vi "Close.vi"(8 "error in (no error)":errorcluster, 11 "DiscoveryService in":refnum<class "NodeDiscovery.lvclass">) -> (0 "error out":errorcluster)   [LabVIEW 2020, in "Vecto.lvlib" / "NodeDiscovery.lvclass"]
uses:
  NodeDiscovery.lvclass
  NodeDiscovery.lvclass/NodeDiscovery.ctl
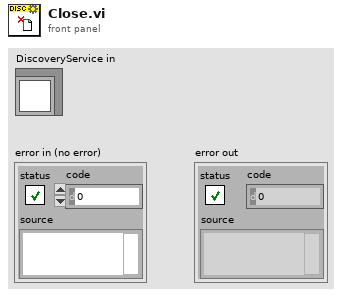
[diagram p1: front panel]
types:
  T1 = typedef "Vecto.lvlib/NodeDiscovery.lvclass/Incoming Events.ctl" = cluster{"Close":refnum<user-event>, "Update Service":refnum<user-event>, "Update Status":refnum<user-event>, "Remove Service":refnum<user-event>}
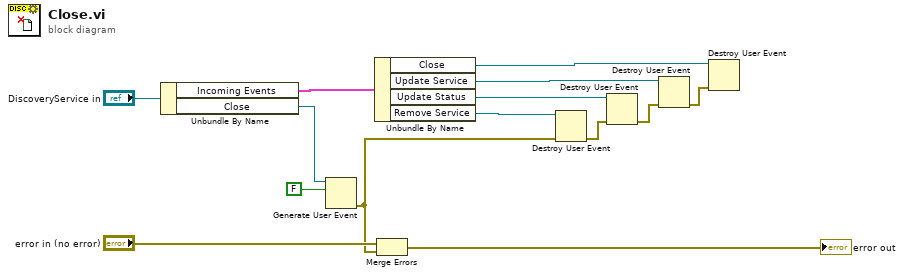
[diagram p0: block diagram]
diagram:
  n1 = Unbundle By Name("DiscoveryService in") -> ("Incoming Events"=w11:T1, "Close"=w13:refnum<user-event>)
  n2 = Generate User Event(user event=w13, event data cluster=FALSE ("event data")) -> (error out=w1:errorcluster)  [unwired: 2 in, 1 out]
  n3 = Unbundle By Name(w11) -> ("Close"=w8:refnum<user-event>, "Update Service"=w9:refnum<user-event>, "Update Status"=w10:refnum<user-event>, "Remove Service"=w4:refnum<user-event>)
  n4 = Merge Errors("error in (no error)", w1) -> (→"error out":errorcluster)
  n5 = Destroy User Event(user event=w4, error in=w1) -> (error out=w3:errorcluster)
  n6 = Destroy User Event(user event=w10, error in=w3) -> (error out=w7:errorcluster)
  n7 = Destroy User Event(user event=w9, error in=w7) -> (error out=w6:errorcluster)
  n8 = Destroy User Event(user event=w8, error in=w6) -> ()  [unwired: 1 out]
